vi "Control Experiment FGV.vi"(6 "Function":enum16{"read", "write"}(ring), 8 "error in (no error)":errorcluster, 11 "Control Experiment.lvclass":refnum<class "Control Experiment.lvclass">) -> (0 "error out":errorcluster, 3 "Control Experiment.lvclass out":refnum<class "Control Experiment.lvclass">)   [LabVIEW 2016, in "Control Experiment.lvclass"]
uses:
  Control Experiment.lvclass
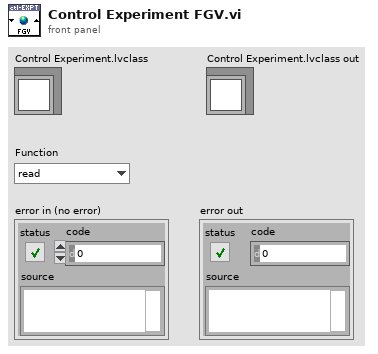
[diagram p1: front panel]
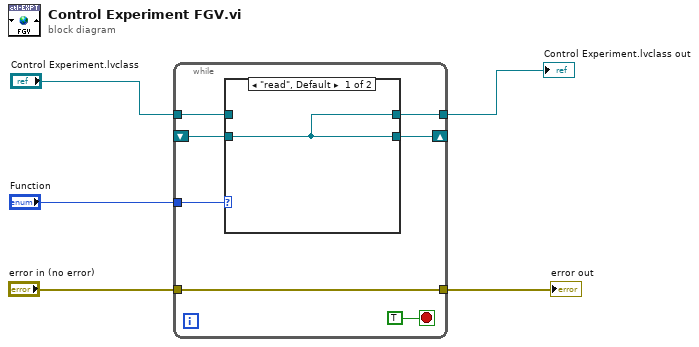
[diagram p0: block diagram]
diagram:
  n1 = while {
    tunnel: "Control Experiment.lvclass" -> [w8]
    tunnel: "error in (no error)" -> [w12]
    tunnel: [w12] -> w5
    tunnel: [w7] -> w1
    shift-right: [w9] -> _
    shift-left: _ -> [w6]
    tunnel: "Function" -> [w10]
    stop <- TRUE stop-if-true
    n2 = case shown="\"read\", Default" w10 {
      tunnel: [w13 w14] -> w9
      tunnel: w8 -> [_ w14]
      tunnel: [w13 w14] -> w7
      tunnel: w6 -> [w13 _]
      frame "read", Default {
      }
      frame "write" {
      }
    }
  }
  "error out" <- w5
  "Control Experiment.lvclass out" <- w1
